vi "Com_SECS Equipment _Message Data Decoding.vi"(8 "error in":errorcluster, 11 "Message Data In":u8[](array[numeric])) -> (0 "error out":errorcluster, 2 "Error?":bool, 3 "Message Data Out":T1[](array[typedef]))   [LabVIEW 2016]
uses:
  Data Def/Com_SECS Equipment _Message Data.ctl
  Data Def/Com_SECS Equipment _Data Item Format.ctl
  Data Def/Com_SECS Equipment _Format Code.ctl
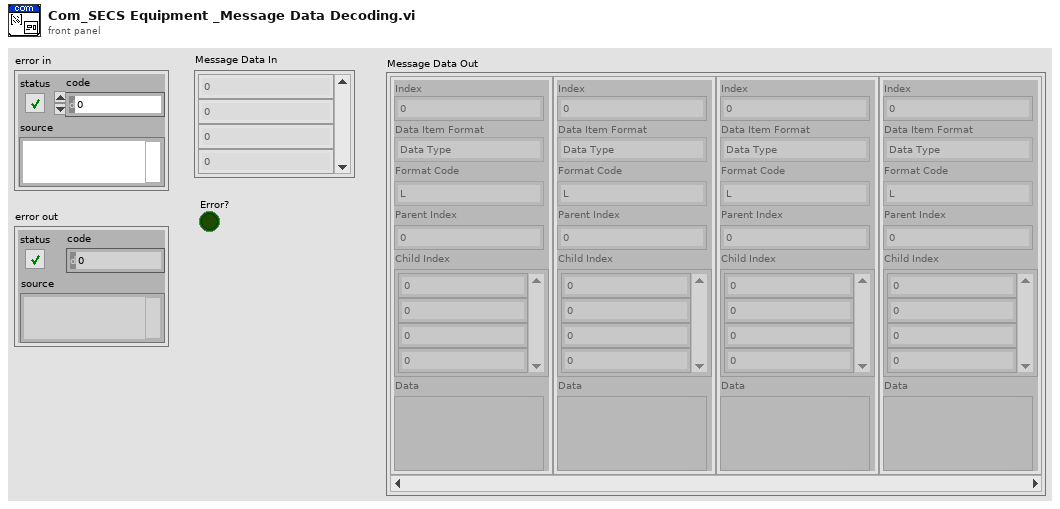
[diagram p1: front panel]
types:
  T1 = typedef "Com_SECS Equipment _Message Data.ctl" = cluster{"Index":i32, "Data Item Format":T2, "Format Code":T3, "Parent Index":i32, "Child Index":i32[], "Data":variant}
  T2 = typedef "Com_SECS Equipment _Data Item Format.ctl" = enum16{"Data Type", "Value"}
  T3 = typedef "Com_SECS Equipment _Format Code.ctl" = enum16{"L", "A", "B", "Boolean", "J", "I1", "I2", "I4", "I8", "U1", "U2", "U4", "U8", "F4", "F8", "Char"}
  T4 = cluster{"Index":i32, "Data Item Format":T2, "Count":i32, "Error?":bool, "Data Length":u32, "Format Code":T3, "Data Index":i32, "Parent Index":i32[], "Correct":bool}
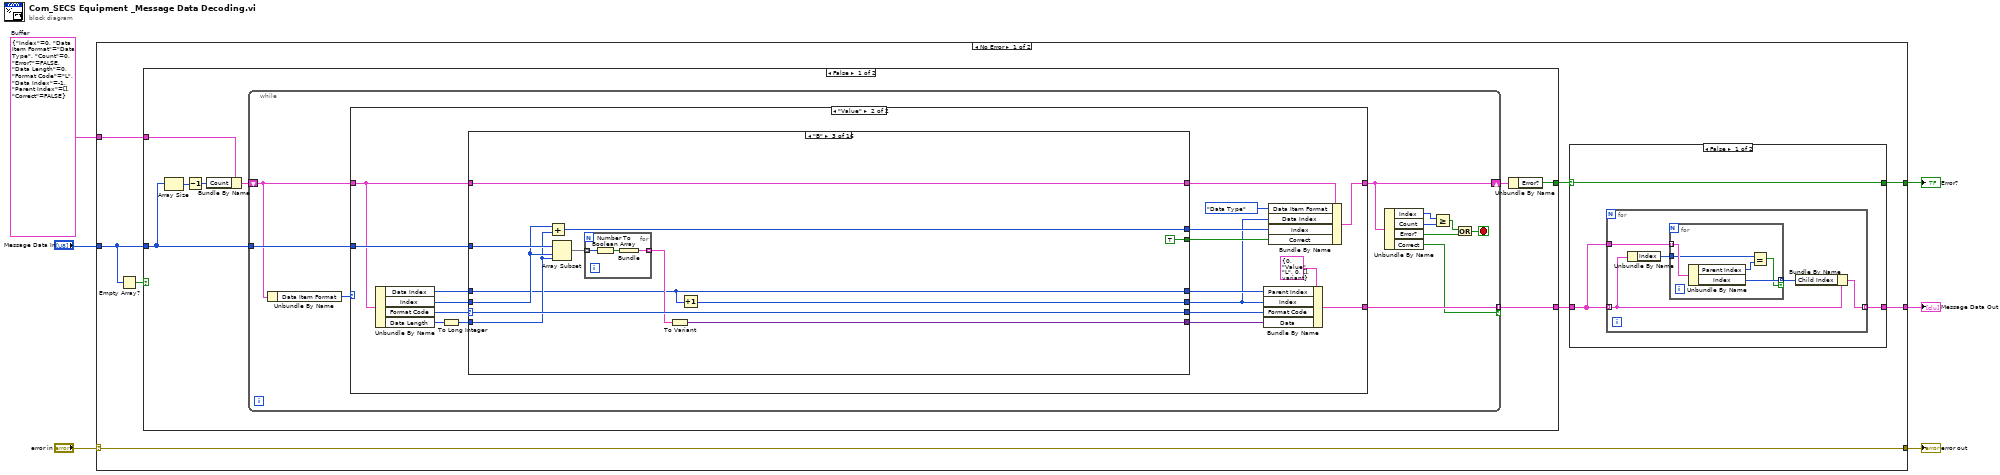
[diagram p0: block diagram]
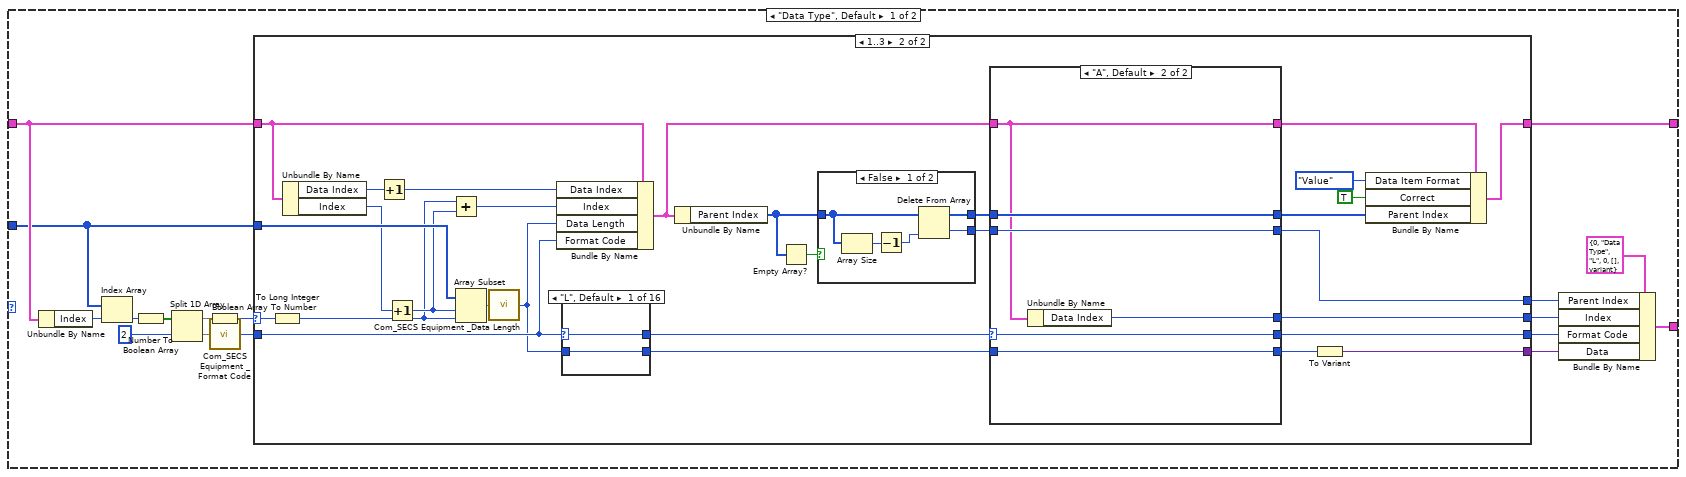
[diagram p3: hidden frame]
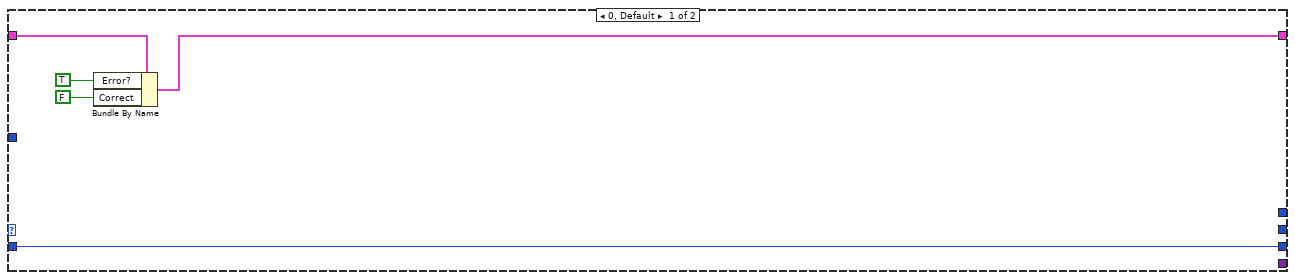
[diagram p4: hidden frame]
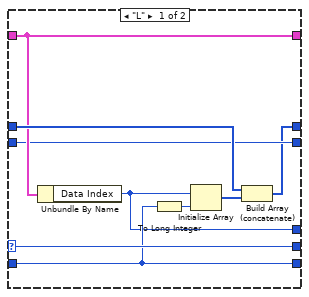
[diagram p5: hidden frame]
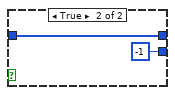
[diagram p6: hidden frame]
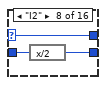
[diagram p13: hidden frame]
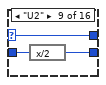
[diagram p14: hidden frame]
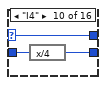
[diagram p15: hidden frame]
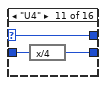
[diagram p16: hidden frame]
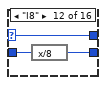
[diagram p17: hidden frame]
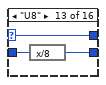
[diagram p18: hidden frame]
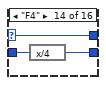
[diagram p19: hidden frame]
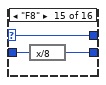
[diagram p20: hidden frame]
diagram:
  w2 = T4 {"Index"=0, "Data Item Format"=enum."Data Type", "Count"=0, "Error?"=FALSE, "Data Length"=0, "Format Code"=enum."L", "Data Index"=-1, "Parent Index"=[], "Correct"=FALSE}  # Buffer
  n1 = case shown="No Error" "error in" {
    selector: "error in" -> [w13 w443]
    tunnel: [w13 w443] -> w3
    tunnel: "Message Data In" -> [w12 _]
    tunnel: [w8 _] -> w4
    tunnel: w2 -> [w11 _]
    tunnel: [w7 TRUE] -> w1
    frame No Error {
      n2 = Empty Array?(array=w12) -> (empty?=w14:bool)
      n3 = case shown="False" w14 {
        tunnel: w12 -> [w36 _]
        tunnel: [w33 _] -> w9
        tunnel: w11 -> [w32 _]
        tunnel: [w30 TRUE ("Error?")] -> w10
        frame False {
          n4 = Array Size(array=w36) -> (size(s)=w35:i32)
          n5 = Decrement(x=w35) -> (x-1=w34:i32)
          n6 = Bundle By Name(cluster=w32, "Count"=w34) -> (w37:T4)
          n7 = while {
            tunnel: w36 -> [w47]
            shift-right: [w44] -> w31
            shift-left: w37 -> [w46]
            tunnel: [w45] -> w33 mode=indexing if=w40
            stop <- w38 stop-if-true
            n8 = Unbundle By Name(w46) -> ("Data Item Format"=w48:T2)
            n9 = case shown="\"Value\"" w48 {
              tunnel: w47 -> [w53 w179]
              tunnel: w46 -> [w58 w166]
              tunnel: [w56 w176] -> w44
              tunnel: [w54 w172] -> w45
              frame "Data Type", Default {
                n10 = Unbundle By Name(w58) -> ("Index"=w65:i32)
                n11 = Index Array(array=w53, index=w65) -> (element=w64:u8)
                n12 = Number To Boolean Array(number=w64) -> (Boolean array=w63:bool[])
                n13 = Split 1D Array(array=w63, index=2) -> (first subarray=w61:bool[], second subarray=w60:bool[])
                n14 = Boolean Array To Number(Boolean array=w61) -> (number=w59:u32)
                n15 = call "Com_SECS Equipment _Format Code.vi"("Formay Code"=w60) -> ("Format Code"=w57:T3)
                n16 = case shown="1..3" w59 {
                  selector: w59 -> [_ w99]
                  tunnel: w58 -> [w70 w87]
                  tunnel: [w69 w78] -> w56
                  tunnel: w57 -> [w68 w92]
                  tunnel: [w68 w81] -> w55
                  tunnel: w53 -> [_ w98]
                  tunnel: [_ w75] -> w51
                  tunnel: [_ w74] -> w50
                  tunnel: [_ w71] -> w49
                  frame 0, Default {
                    n17 = Bundle By Name(cluster=w70, "Error?"=TRUE, "Correct"=FALSE) -> (w69:T4)
                  }
                  frame 1..3 {
                    n18 = To Long Integer(number=w99) -> (32bit integer=w93:i32)
                    n19 = Unbundle By Name(w87) -> ("Data Index"=w90:i32, "Index"=w97:i32)
                    n20 = Increment(x=w90) -> (x+1=w89:i32)
                    n21 = Increment(x=w97) -> (x+1=w95:i32)
                    n22 = Add(x=w93, y=w95) -> (x+y=w94:i32)
                    n23 = Array Subset(array=w98, index=w95, length=w93) -> (w96:u8[])
                    n24 = call "Com_SECS Equipment _Data Length.vi"("Data Length U8 []"=w96) -> ("Data Length"=w91:u32)
                    n25 = Bundle By Name(cluster=w87, "Data Index"=w89, "Index"=w94, "Data Length"=w91, "Format Code"=w92) -> (w73:T4)
                    n26 = case shown="\"L\", Default" w92 {
                      selector: w92 -> [w123 w125 w127 w129 w131 w133 w135 w138 w141 w144 w147 w150 w153 w156 w159 w162]
                      tunnel: [w123 w125 w127 w129 w131 w133 w135 w138 w141 w144 w147 w150 w153 w156 w159 w162] -> w85
                      tunnel: w91 -> [w122 w124 w126 w128 w130 w132 w134 w137 w140 w143 w146 w149 w152 w155 w158 w161]
                      tunnel: [w122 w124 w126 w128 w130 w132 w134 w136 w139 w142 w145 w148 w151 w154 w157 w160] -> w84
                      frame "L", Default {
                      }
                      frame "A" {
                      }
                      frame "B" {
                      }
                      frame "Boolean" {
                      }
                      frame "J" {
                      }
                      frame "I1" {
                      }
                      frame "U1" {
                      }
                      frame "I2" {
                        n27 = expression code="x/2"(w137) -> (w136:u32)
                      }
                      frame "U2" {
                        n28 = expression code="x/2"(w140) -> (w139:u32)
                      }
                      frame "I4" {
                        n29 = expression code="x/4"(w143) -> (w142:u32)
                      }
                      frame "U4" {
                        n30 = expression code="x/4"(w146) -> (w145:u32)
                      }
                      frame "I8" {
                        n31 = expression code="x/8"(w149) -> (w148:u32)
                      }
                      frame "U8" {
                        n32 = expression code="x/8"(w152) -> (w151:u32)
                      }
                      frame "F4" {
                        n33 = expression code="x/4"(w155) -> (w154:u32)
                      }
                      frame "F8" {
                        n34 = expression code="x/8"(w158) -> (w157:u32)
                      }
                      frame "Char" {
                        n35 = expression code="x/2"(w161) -> (w160:u32)
                      }
                    }
                    n36 = Unbundle By Name(w73) -> ("Parent Index"=w86:i32[])
                    n37 = Empty Array?(array=w86) -> (empty?=w88:bool)
                    n38 = case shown="False" w88 {
                      tunnel: w86 -> [w119 w121]
                      tunnel: [w117 w121] -> w83
                      tunnel: [w116 -1 ("Numeric")] -> w82
                      frame False {
                        n39 = Array Size(array=w119) -> (size(s)=w118:i32)
                        n40 = Decrement(x=w118) -> (x-1=w115:i32)
                        n41 = Delete From Array(array=w119, index=w115) -> (deleted portion=w116:i32, array with subset deleted=w117:i32[])  [unwired: 1 in]
                      }
                      frame True {
                      }
                    }
                    n42 = case shown="\"A\", Default" w85 {
                      selector: w85 -> [w108 w113]
                      tunnel: w84 -> [w107 w114]
                      tunnel: w83 -> [w105 w112]
                      tunnel: w82 -> [w102 w111]
                      tunnel: w73 -> [w103 w110]
                      tunnel: [w108 w113] -> w81
                      tunnel: [w107 w114] -> w72
                      tunnel: [w103 w110] -> w80
                      tunnel: [w101 w112] -> w79
                      tunnel: [w102 w111] -> w74
                      tunnel: [w100 w109] -> w75
                      frame "L" {
                        n43 = Unbundle By Name(w103) -> ("Data Index"=w100:i32)
                        n44 = To Long Integer(number=w107) -> (32bit integer=w106:i32)
                        n45 = Initialize Array(w100, w106) -> (w104:i32[])
                        n46 = Build Array (concatenate)(w105, w104) -> (w101:i32[])
                      }
                      frame "A", Default {
                        n47 = Unbundle By Name(w110) -> ("Data Index"=w109:i32)
                      }
                    }
                    n48 = To Variant(anything=w72) -> (Variant=w71:variant)
                    n49 = Bundle By Name(cluster=w80, "Data Item Format"=Com_SECS_Equipment__Data_Item_Format."Value", "Correct"=TRUE, "Parent Index"=w79) -> (w78:T4)
                  }
                }
                n50 = Bundle By Name(cluster=T1 {"Index"=0, "Data Item Format"=enum."Data Type", "Format Code"=enum."L", "Parent Index"=0, "Child Index"=[], "Data"=variant} ("Message Data"), "Parent Index"=w50, "Index"=w51, "Format Code"=w55, "Data"=w49) -> (w54:T1)
              }
              frame "Value" {
                n51 = Unbundle By Name(w166) -> ("Data Index"=w168:i32, "Index"=w171:i32, "Format Code"=w180:T3, "Data Length"=w175:u32)
                n52 = To Long Integer(number=w175) -> (32bit integer=w174:i32)
                n53 = case shown="\"B\"" w180 {
                  selector: w180 -> [w186 w199 w211 w226 w237 w249 w260 w274 w295 w316 w337 w358 w379 w400 w421 w440]
                  tunnel: w179 -> [_ w197 w209 w224 w235 w247 w258 w272 w293 w314 w335 w356 w377 w398 w419 w438]
                  tunnel: w166 -> [w187 w198 w210 w225 w236 w248 w259 w273 w294 w315 w336 w357 w378 w399 w420 w439]
                  tunnel: [w187 w198 w210 w225 w236 w248 w259 w273 w294 w315 w336 w357 w378 w399 w420 w439] -> w177
                  tunnel: w174 -> [w182 w194 w207 w222 w233 w245 w256 w270 w291 w312 w333 w354 w375 w396 w417 w436]
                  tunnel: [w186 w199 w211 w226 w237 w249 w260 w274 w295 w316 w337 w358 w379 w400 w421 w440] -> w173
                  tunnel: w171 -> [w185 w195 w208 w223 w234 w246 w257 w271 w292 w313 w334 w355 w376 w397 w418 w437]
                  tunnel: [w183 w192 w206 w221 w232 w244 w255 w269 w290 w311 w332 w353 w374 w395 w416 w433] -> w170
                  tunnel: w168 -> [w181 w188 w203 w218 w229 w240 w252 w262 w283 w304 w325 w346 w367 w388 w409 w431]
                  tunnel: [w181 w189 w201 w215 w228 w239 w251 w261 w282 w303 w324 w345 w366 w387 w408 w430] -> w163
                  tunnel: [w181 w188 w203 w218 w229 w240 w252 w262 w283 w304 w325 w346 w367 w388 w409 w431] -> w167
                  tunnel: [w185 w191 w202 w216 w230 w241 w253 w264 w285 w306 w327 w348 w369 w390 w411 w432] -> w165
                  tunnel: [FALSE TRUE TRUE TRUE TRUE TRUE TRUE TRUE TRUE TRUE TRUE TRUE TRUE TRUE TRUE TRUE] -> w164
                  frame "L" {
                    n54 = To Variant(anything=w182) -> (Variant=w183:variant)
                  }
                  frame "A", Default {
                    n55 = Add(x=w195, y=w194) -> (x+y=w191:i32)
                    n56 = Array Subset(array=w197, index=w195, length=w194) -> (w196:u8[])
                    n57 = Byte Array To String(unsigned byte array=w196) -> (string=w193:string)
                    n58 = To Variant(anything=w193) -> (Variant=w192:variant)
                    n59 = Increment(x=w188) -> (x+1=w189:i32)
                  }
                  frame "B" {
                    n60 = Add(x=w208, y=w207) -> (x+y=w202:i32)
                    n61 = Array Subset(array=w209, index=w208, length=w207) -> (w205:u8[])
                    n62 = for {
                      tunnel: w205 -> [w214] mode=indexing
                      tunnel: [w212] -> w204 mode=indexing
                      n63 = Number To Boolean Array(number=w214) -> (Boolean array=w213:bool[])
                      n64 = Bundle("Boolean array"=w213) -> (w212:cluster{"Boolean array":bool[]})  [unwired: 1 in]
                    }
                    n65 = To Variant(anything=w204) -> (Variant=w206:variant)
                    n66 = Increment(x=w203) -> (x+1=w201:i32)
                  }
                  frame "Boolean" {
                    n67 = Add(x=w223, y=w222) -> (x+y=w216:i32)
                    n68 = Array Subset(array=w224, index=w223, length=w222) -> (w220:u8[])
                    n69 = Not Equal To 0?(x=w220) -> (x != 0?=w219:bool[])
                    n70 = To Variant(anything=w219) -> (Variant=w221:variant)
                    n71 = Increment(x=w218) -> (x+1=w215:i32)
                  }
                  frame "J" {
                    n72 = Array Subset(array=w235, index=w234, length=w233) -> (w231:u8[])
                    n73 = Add(x=w234, y=w233) -> (x+y=w230:i32)
                    n74 = To Variant(anything=w231) -> (Variant=w232:variant)
                    n75 = Increment(x=w229) -> (x+1=w228:i32)
                  }
                  frame "I1" {
                    n76 = Add(x=w246, y=w245) -> (x+y=w241:i32)
                    n77 = Array Subset(array=w247, index=w246, length=w245) -> (w243:u8[])
                    n78 = To Byte Integer(number=w243) -> (8bit integer=w242:i8[])
                    n79 = To Variant(anything=w242) -> (Variant=w244:variant)
                    n80 = Increment(x=w240) -> (x+1=w239:i32)
                  }
                  frame "U1" {
                    n81 = Add(x=w257, y=w256) -> (x+y=w253:i32)
                    n82 = Array Subset(array=w258, index=w257, length=w256) -> (w254:u8[])
                    n83 = To Variant(anything=w254) -> (Variant=w255:variant)
                    n84 = Increment(x=w252) -> (x+1=w251:i32)
                  }
                  frame "I2" {
                    n85 = Add(x=w271, y=w270) -> (x+y=w264:i32)
                    n86 = Array Subset(array=w272, index=w271, length=w270) -> (w266:u8[])
                    n87 = Array Size(array=w266) -> (size(s)=w268:i32)
                    n88 = expression code="x/2"(w268) -> (w267:i32)
                    n89 = for {
                      N: w267 -> [_]
                      tunnel: w266 -> [w281]
                      tunnel: [w275] -> w265 mode=indexing
                      i -> [w280]
                      n90 = expression code="x*2"(w280) -> (w279:i32)
                      n91 = Index Array(array=w281, index #1=w279) -> (element #1=w277:u8, element #2=w278:u8)  [unwired: 1 in]
                      n92 = Join Numbers(hi=w277, lo=w278) -> ((hi.lo)=w276:u16)
                      n93 = To Word Integer(number=w276) -> (16bit integer=w275:i16)
                    }
                    n94 = To Variant(anything=w265) -> (Variant=w269:variant)
                    n95 = Increment(x=w262) -> (x+1=w261:i32)
                  }
                  frame "U2" {
                    n96 = Add(x=w292, y=w291) -> (x+y=w285:i32)
                    n97 = Array Subset(array=w293, index=w292, length=w291) -> (w287:u8[])
                    n98 = Array Size(array=w287) -> (size(s)=w289:i32)
                    n99 = expression code="x/2"(w289) -> (w288:i32)
                    n100 = for {
                      N: w288 -> [_]
                      tunnel: w287 -> [w302]
                      tunnel: [w296] -> w286 mode=indexing
                      i -> [w301]
                      n101 = expression code="x*2"(w301) -> (w300:i32)
                      n102 = Index Array(array=w302, index #1=w300) -> (element #1=w298:u8, element #2=w299:u8)  [unwired: 1 in]
                      n103 = Join Numbers(hi=w298, lo=w299) -> ((hi.lo)=w297:u16)
                      n104 = To Unsigned Word Integer(number=w297) -> (unsigned 16bit integer=w296:u16)
                    }
                    n105 = To Variant(anything=w286) -> (Variant=w290:variant)
                    n106 = Increment(x=w283) -> (x+1=w282:i32)
                  }
                  frame "I4" {
                    n107 = Add(x=w313, y=w312) -> (x+y=w306:i32)
                    n108 = Array Subset(array=w314, index=w313, length=w312) -> (w308:u8[])
                    n109 = Array Size(array=w308) -> (size(s)=w310:i32)
                    n110 = expression code="x/4"(w310) -> (w309:i32)
                    n111 = for {
                      N: w309 -> [_]
                      tunnel: w308 -> [w323]
                      tunnel: [w317] -> w307 mode=indexing
                      i -> [w322]
                      n112 = expression code="x*4"(w322) -> (w321:i32)
                      n113 = Array Subset(array=w323, index=w321, length=4) -> (w319:u8[])
                      n114 = Type Cast(type=0, x=w319) -> (*(type *) &x=w317:i32)
                    }
                    n115 = To Variant(anything=w307) -> (Variant=w311:variant)
                    n116 = Increment(x=w304) -> (x+1=w303:i32)
                  }
                  frame "U4" {
                    n117 = Add(x=w334, y=w333) -> (x+y=w327:i32)
                    n118 = Array Subset(array=w335, index=w334, length=w333) -> (w329:u8[])
                    n119 = Array Size(array=w329) -> (size(s)=w331:i32)
                    n120 = expression code="x/4"(w331) -> (w330:i32)
                    n121 = for {
                      N: w330 -> [_]
                      tunnel: w329 -> [w344]
                      tunnel: [w338] -> w328 mode=indexing
                      i -> [w343]
                      n122 = expression code="x*4"(w343) -> (w342:i32)
                      n123 = Array Subset(array=w344, index=w342, length=4) -> (w340:u8[])
                      n124 = Type Cast(type=u32 0, x=w340) -> (*(type *) &x=w338:u32)
                    }
                    n125 = To Variant(anything=w328) -> (Variant=w332:variant)
                    n126 = Increment(x=w325) -> (x+1=w324:i32)
                  }
                  frame "I8" {
                    n127 = Add(x=w355, y=w354) -> (x+y=w348:i32)
                    n128 = Array Subset(array=w356, index=w355, length=w354) -> (w350:u8[])
                    n129 = Array Size(array=w350) -> (size(s)=w352:i32)
                    n130 = expression code="x/8"(w352) -> (w351:i32)
                    n131 = for {
                      N: w351 -> [_]
                      tunnel: w350 -> [w365]
                      tunnel: [w359] -> w349 mode=indexing
                      i -> [w364]
                      n132 = expression code="x*8"(w364) -> (w363:i32)
                      n133 = Array Subset(array=w365, index=w363, length=8) -> (w361:u8[])
                      n134 = Type Cast(type=i64 0, x=w361) -> (*(type *) &x=w359:i64)
                    }
                    n135 = To Variant(anything=w349) -> (Variant=w353:variant)
                    n136 = Increment(x=w346) -> (x+1=w345:i32)
                  }
                  frame "U8" {
                    n137 = Add(x=w376, y=w375) -> (x+y=w369:i32)
                    n138 = Array Subset(array=w377, index=w376, length=w375) -> (w371:u8[])
                    n139 = Array Size(array=w371) -> (size(s)=w373:i32)
                    n140 = expression code="x/8"(w373) -> (w372:i32)
                    n141 = for {
                      N: w372 -> [_]
                      tunnel: w371 -> [w386]
                      tunnel: [w380] -> w370 mode=indexing
                      i -> [w385]
                      n142 = expression code="x*8"(w385) -> (w384:i32)
                      n143 = Array Subset(array=w386, index=w384, length=8) -> (w382:u8[])
                      n144 = Type Cast(type=u64 0, x=w382) -> (*(type *) &x=w380:u64)
                    }
                    n145 = To Variant(anything=w370) -> (Variant=w374:variant)
                    n146 = Increment(x=w367) -> (x+1=w366:i32)
                  }
                  frame "F4" {
                    n147 = Add(x=w397, y=w396) -> (x+y=w390:i32)
                    n148 = Array Subset(array=w398, index=w397, length=w396) -> (w392:u8[])
                    n149 = Array Size(array=w392) -> (size(s)=w394:i32)
                    n150 = expression code="x/4"(w394) -> (w393:i32)
                    n151 = for {
                      N: w393 -> [_]
                      tunnel: w392 -> [w407]
                      tunnel: [w401] -> w391 mode=indexing
                      i -> [w406]
                      n152 = expression code="x*4"(w406) -> (w405:i32)
                      n153 = Array Subset(array=w407, index=w405, length=4) -> (w403:u8[])
                      n154 = Type Cast(type=sgl 0.0, x=w403) -> (*(type *) &x=w401:sgl)
                    }
                    n155 = To Variant(anything=w391) -> (Variant=w395:variant)
                    n156 = Increment(x=w388) -> (x+1=w387:i32)
                  }
                  frame "F8" {
                    n157 = Add(x=w418, y=w417) -> (x+y=w411:i32)
                    n158 = Array Subset(array=w419, index=w418, length=w417) -> (w413:u8[])
                    n159 = Array Size(array=w413) -> (size(s)=w415:i32)
                    n160 = expression code="x/8"(w415) -> (w414:i32)
                    n161 = for {
                      N: w414 -> [_]
                      tunnel: w413 -> [w428]
                      tunnel: [w422] -> w412 mode=indexing
                      i -> [w427]
                      n162 = expression code="x*8"(w427) -> (w426:i32)
                      n163 = Array Subset(array=w428, index=w426, length=8) -> (w424:u8[])
                      n164 = Type Cast(type=0.0, x=w424) -> (*(type *) &x=w422:dbl)
                    }
                    n165 = To Variant(anything=w412) -> (Variant=w416:variant)
                    n166 = Increment(x=w409) -> (x+1=w408:i32)
                  }
                  frame "Char" {
                    n167 = Add(x=w437, y=w436) -> (x+y=w432:i32)
                    n168 = Array Subset(array=w438, index=w437, length=w436) -> (w435:u8[])
                    n169 = Byte Array To String(unsigned byte array=w435) -> (string=w434:string)
                    n170 = To Variant(anything=w434) -> (Variant=w433:variant)
                    n171 = Increment(x=w431) -> (x+1=w430:i32)
                  }
                }
                n172 = Bundle By Name(cluster=T1 {"Index"=0, "Data Item Format"=enum."Value", "Format Code"=enum."L", "Parent Index"=0, "Child Index"=[], "Data"=variant} ("Message Data"), "Parent Index"=w167, "Index"=w163, "Format Code"=w173, "Data"=w170) -> (w172:T1)
                n173 = Bundle By Name(cluster=w177, "Data Item Format"=Com_SECS_Equipment__Data_Item_Format."Data Type", "Data Index"=w163, "Index"=w165, "Correct"=w164) -> (w176:T4)
              }
            }
            n174 = Unbundle By Name(w44) -> ("Index"=w39:i32, "Count"=w43:i32, "Error?"=w41:bool, "Correct"=w40:bool)
            n175 = Greater Or Equal?(x=w39, y=w43) -> (x >= y?=w42:bool)
            n176 = Or(x=w42, y=w41) -> (x .or. y?=w38:bool)
          }
          n177 = Unbundle By Name(w31) -> ("Error?"=w30:bool)
        }
        frame True {
        }
      }
      n178 = case shown="False" w10 {
        selector: w10 -> [w15 w29]
        tunnel: w9 -> [w17 w28]
        tunnel: [w16 w28] -> w8
        tunnel: [w15 w29] -> w7
        frame False {
          n179 = for {
            tunnel: w17 -> [w20] mode=indexing
            tunnel: w17 -> [w22]
            tunnel: [w18] -> w16 mode=indexing
            n180 = Unbundle By Name(w20) -> ("Index"=w21:i32)
            n181 = for {
              tunnel: w22 -> [w27] mode=indexing
              tunnel: w21 -> [w26]
              tunnel: [w24] -> w19 mode=indexing if=w23
              n182 = Unbundle By Name(w27) -> ("Parent Index"=w25:i32, "Index"=w24:i32)
              n183 = Equal?(x=w26, y=w25) -> (x = y?=w23:bool)
            }
            n184 = Bundle By Name(cluster=w20, "Child Index"=w19) -> (w18:T1)
          }
        }
        frame True {
        }
      }
    }
    frame Error {
    }
  }
  "error out" <- w3
  "Error?" <- w1
  "Message Data Out" <- w4
